vi "About.vi"(10 "窗口边界":T1) -> ()   [LabVIEW 2015]
doc: "本VI是为《我和LabVIEW》一书编写的示例。\n关于本书的介绍请参考网页：\nhttp://ruanqizhen.spaces.live.com/blog/cns!5852D4F797C53FB6!4310.entry"
uses:
  <vilib>/Utility/miscctls.llb/LVRectTypeDef.ctl
  user32.dll
panel:
  # "PAM Control Module For Debug\nVer0.1\n\n上海磨智科技有限公司\nShanghai Muzi-Tek Co.,Ltd\n官方网址：www.muzi-tek.com"
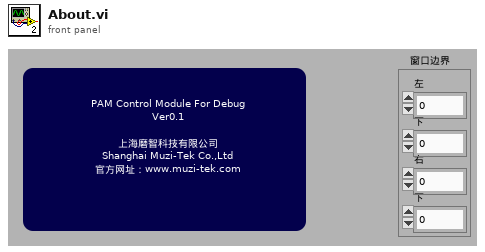
[diagram p1: front panel]
types:
  T1 = typedef "LVRectTypeDef.ctl" = cluster{"Left":i16, "Top":i16, "Right":i16, "Bottom":i16}
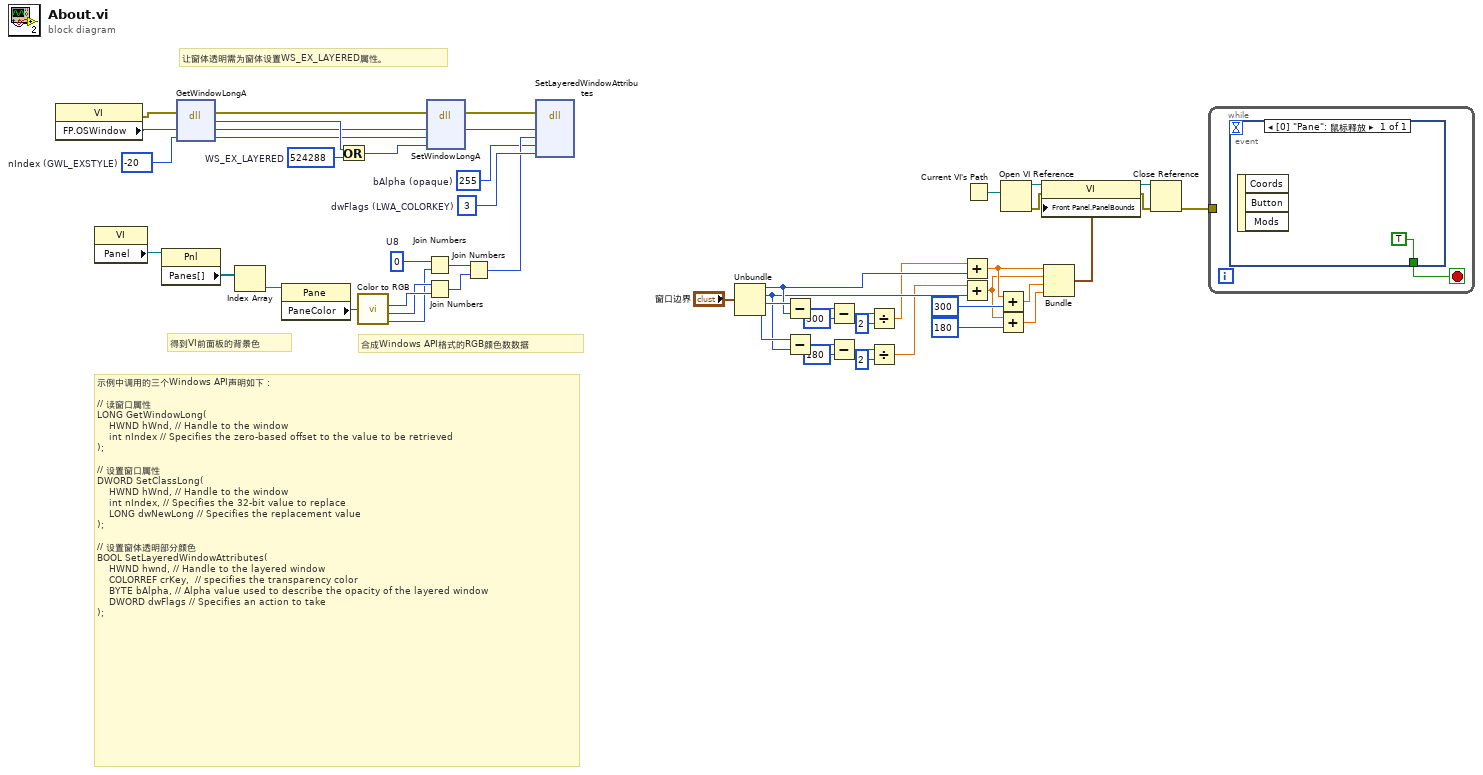
[diagram p0: block diagram]
diagram:
  w13 = 524288  # WS_EX_LAYERED
  w10 = -20  # nIndex (GWL_EXSTYLE)
  w16 = 255  # bAlpha (opaque)
  w17 = u8 0  # U8
  w21 = 3  # dwFlags (LWA_COLORKEY)
  # "示例中调用的三个Windows API声明如下：\n\n// 读窗口属性\nLONG GetWindowLong(      \n    HWND hWnd,\t// Handle to the window\n    int nIndex\t// Specifies the zero-based offset to the value to be retrieved\n);\n\n// 设置窗口属性\nDWORD SetClassLong(      \n    HWND hWnd,\t// Handle to the window\n    int nIndex,\t// Specifies the 32-bit value to replace\n    LONG dwNewLong // Specifies the replacement value\n);\n\n// 设置窗体透明部分颜色\nBOOL SetLayeredWindowAttributes(      \n    HWND hwnd,\t// Handle to the layered window\n    COLORREF crKey,  // specifies the transparency color\n    BYTE bAlpha,\t// Alpha value used to describe the opacity of the layered window\n    DWORD dwFlags\t// Specifies an action to take\n);"
  # "让窗体透明需为窗体设置WS_EX_LAYERED属性。"
  # "合成Windows API格式的RGB颜色数数据"
  # "得到VI前面板的背景色"
  n1 = property class="VI"() -> (error out=w8:errorcluster, "FP.OSWindow"=w12:i32)  [unwired: 2 in, 1 out]
  n2 = property class="VI"() -> ("Panel"=w24:refnum<vi>)  [unwired: 2 in, 2 out]
  n3 = property class="Pnl"(reference=w24) -> ("Panes[]"=w23:refnum<vi>[])  [unwired: 1 in, 2 out]
  n4 = dll-call lib="USER32.DLL" fn="GetWindowLongA" label="getWindowLong"(error in=w8, "handle"=w12, "nIndex"=w10) -> (error out=w7:errorcluster, w14:i32, "handle"=w11:i32, "nIndex"=w9:i32)  [unwired: 2 in, 1 out]
  n5 = Index Array(array=w23) -> (element=w22:refnum<vi>)  [unwired: 1 in]
  n6 = property class="Pane"(reference=w22) -> ("PaneColor"=w4:u32)  [unwired: 1 in, 2 out]
  n7 = Or(x=w14, y=w13) -> (x .or. y?=w15:i32)
  n8 = call <vilib>:"Color to RGB.vi"("Color"=w4) -> ("R"=w3:u8, "G"=w2:u8, "B"=w1:u8)  [unwired: 1 out]
  n9 = Join Numbers(hi=w17, lo=w1) -> ((hi.lo)=w19:u16)
  n10 = Join Numbers(hi=w2, lo=w3) -> ((hi.lo)=w20:u16)
  n11 = dll-call lib="USER32.DLL" fn="SetWindowLongA" label="SetWindowLong"(error in=w7, "handle"=w11, "nIndex"=w9, "dwNewLong"=w15) -> (error out=w6:errorcluster, "handle"=w5:i32)  [unwired: 4 in, 2 out]
  n12 = Join Numbers(hi=w19, lo=w20) -> ((hi.lo)=w18:u32)
  n13 = dll-call lib="USER32.DLL" fn="SetLayeredWindowAttributes" label="SetLayerdWindowAttributs"(error in=w6, "handle"=w5, "crkey"=w18, "bAlpha"=w16, "dwFlags"=w21) -> ()  [unwired: 6 in, 3 out]
  n14 = Unbundle("窗口边界") -> ("Left"=w37:i16, "Top"=w35:i16, "Right"=w38:i16, "Bottom"=w36:i16)
  n15 = Subtract(x=w38, y=w37) -> (x-y=w34:i16)
  n16 = Subtract(x=w36, y=w35) -> (x-y=w32:i16)
  n17 = Subtract(x=w34, y=i16 300) -> (x-y=w30:i16)
  n18 = Subtract(x=w32, y=i16 180) -> (x-y=w29:i16)
  n19 = Divide(x=w30, y=i16 2) -> (x/y=w26:dbl)
  n20 = Divide(x=w29, y=i16 2) -> (x/y=w25:dbl)
  n21 = Add(x=w26, y=w37) -> (x+y=w44:dbl)
  n22 = Add(x=w25, y=w35) -> (x+y=w43:dbl)
  n23 = Current VI's Path() -> (path=w52:path)
  n24 = Add(x=w44, y=i16 300) -> (x+y=w42:dbl)
  n25 = Add(x=w43, y=i16 180) -> (x+y=w41:dbl)
  n26 = Open VI Reference(vi path=w52) -> (vi reference=w51:refnum<vi>, error out=w50:errorcluster)  [unwired: 5 in]
  n27 = Bundle(w44, w43, w42, w41) -> (w40:cluster{dbl, dbl, dbl, dbl})  [unwired: 1 in]
  n28 = property class="VI"(reference=w51, error in=w50, "Front Panel.PanelBounds"=w40) -> (reference out=w48:refnum<vi>, error out=w49:errorcluster)
  n29 = Close Reference(reference=w48, error in (no error)=w49) -> (error out=w39:errorcluster)
  n30 = while {
    tunnel: w39 -> [_]
    stop <- w53 stop-if-true
    n31 = event shown="[0] \"Pane\": 鼠标释放" {
      selector: _ -> [_]
      dyn-events: _ -> [_]
      timeout: _ -> [_]
      tunnel: [TRUE] -> w53
      event Mouse Up {
        n32 = event-data() -> ()  [unwired: 4 out]
      }
    }
  }
